vi "string -- format sweep table string.vi"(9 "ITC set temperature":dbl, 10 "date string Array":string[](array[string])=["Fri, Mar 07, 2014   :   11:06 AM", "Fri, Mar 07, 2014   :   3:06 PM"], 11 "Sweep Table":dbl[][](array[numeric])=[[70.0, 240.0, 1000.0], [0.0, 0.0, 0.0], [0.0, 0.0, 0.0], [0.0, 0.0, 0.0], [0.0, 0.0, 0.0], [0.0, 0.0, 0.0], [0.0, 0.0, 0.0], [0.0, 0.0, 0.0], [0.0, 0.0, 0.0], [0.0, 0.0, 0.0], [0.0, 0.0, 0.0], [0.0, 0.0, 0.0], [0.0, 0.0, 0.0], [0.0, 0.0, 0.0], [0.0, 0.0, 0.0], [70.0, 0.0, 0.0]]) -> (0 "string out":string)   [LabVIEW 2015]
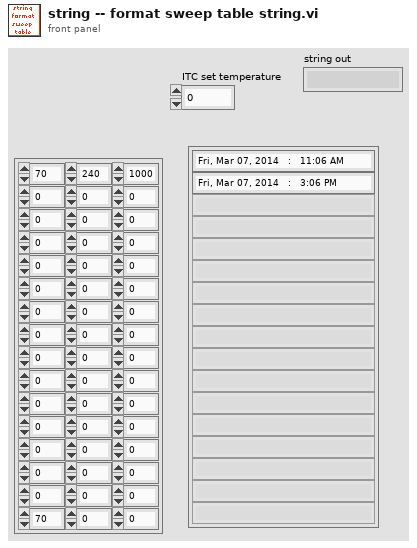
[diagram p1: front panel]
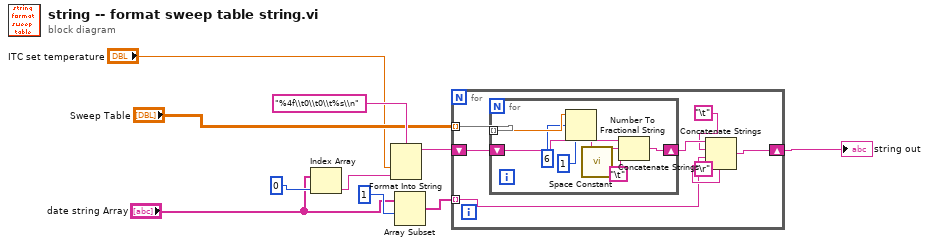
[diagram p0: block diagram]
diagram:
  n1 = Index Array(array="date string Array", index=0) -> (element=w7:string)
  n2 = Format Into String(format string="%4f\\t0\\t0\\t%s\\n" ("action"), "ITC set temperature", w7) -> (resulting string=w6:string)  [unwired: 2 in, 1 out]
  n3 = Array Subset(array="date string Array", index=1) -> (w4:string[])  [unwired: 1 in]
  n4 = for {
    tunnel: "Sweep Table" -> [w17] mode=indexing
    shift-right: [w13] -> w10
    shift-left: w6 -> [w16]
    tunnel: w4 -> [w12] mode=indexing
    n5 = for {
      tunnel: w17 -> [w24] mode=indexing
      shift-right: [w23] -> w15
      shift-left: w16 -> [w22]
      n6 = Number To Fractional String(number=w24, width (-)=i16 6 ("precision (6)"), precision (6)=i16 1) -> (F-format string=w21:string)  [unwired: 1 in]
      n7 = call <vilib>:"Space Constant.vi"() -> ()  [unwired: 1 out]
      n8 = Concatenate Strings(w22, w21, "\t") -> (w23:string)
    }
    n9 = Concatenate Strings(w15, "\t", w12, "\r") -> (w13:string)
  }
  "string out" <- w10
